vi "Ultimate Tab Control.vi"() -> ()   [LabVIEW 2020]
panel:
  in  "button name (\"OK\")":string
  in  "stop":bool
  in  "Page 5":bool
  in  "Radio Buttons":enum32{"Page 1", "Page 2", "Page 3", "Page 4"}(radio)=enum."Page 3"
  in  "Tab Control":T1(tab)
  in  "DOWN":bool
  in  "UP":bool
  out "DOWN":bool
  out "UP":bool
  in  "Rotation":enum32{"Left", "Neutral", "Right"}(radio)=enum."Neutral"
  in  "Slide":dbl(slide) scale=0.0..10.0
  out "Gauge":dbl(knob) scale=0.0..10.0
  in  "PRESS":bool
  out "Waveform Chart":dbl(graph)=1.524663471811628
  # "Notice that the stop button\nis under shadowed.\nThis means it is common to\nall pages of the tab control.\n\nIf it only needs to be visible \non three of the pages use a\nvisibility property node on the block diagram and place a constant true or false on each page."
  # "IF YOU NOTICE THE NEXT\nTIME YOU ARE IN EDIT MODE\nTHAT THE RADIO BUTTONS\nDO NOT CONTROL THE TABS.\n\nTHIS MEANS IN EDIT MODE, MAKE THE \nTABS FOR THE CONTROL VISIBLE\nIN ORDER TO TAB THROUGH THE PAGES."
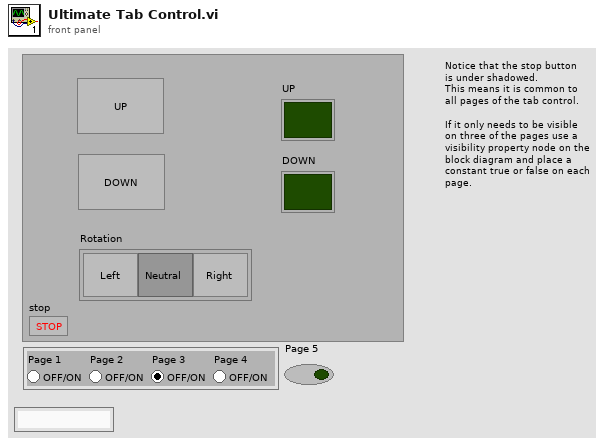
[diagram p1: front panel]
types:
  T1 = enum32{"Page 1", "Page 2", "Page 3", "Page 4", "Page 5"}
  T2 = enum8{"Enabled", "Disabled", "Disabled and Grayed Out"}
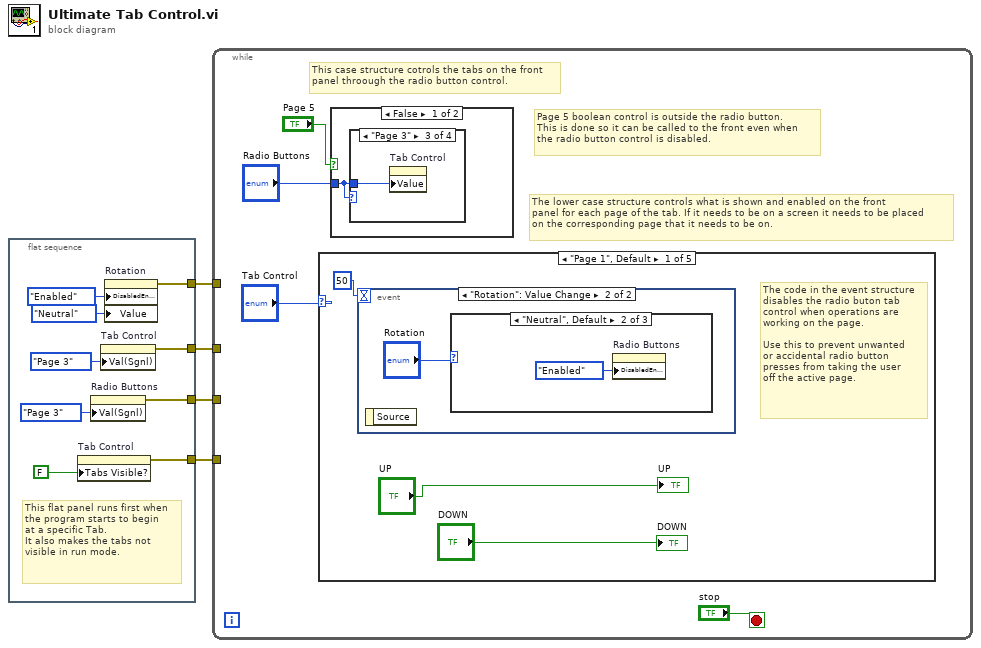
[diagram p0: block diagram]
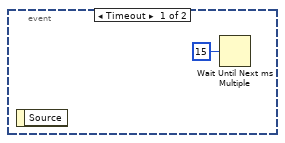
[diagram p2: hidden frame]
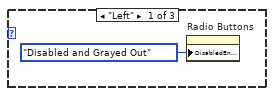
[diagram p3: hidden frame]
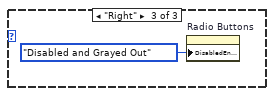
[diagram p4: hidden frame]
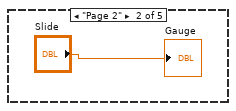
[diagram p5: hidden frame]
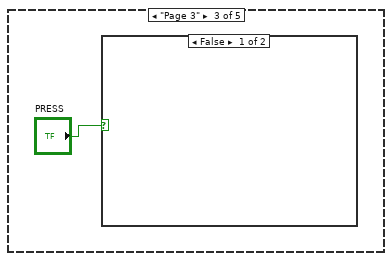
[diagram p6: hidden frame]
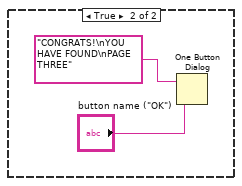
[diagram p7: hidden frame]
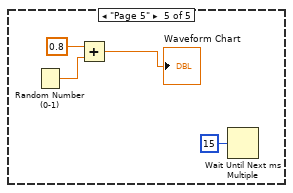
[diagram p9: hidden frame]
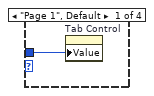
[diagram p10: hidden frame]
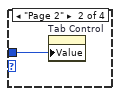
[diagram p11: hidden frame]
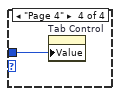
[diagram p12: hidden frame]
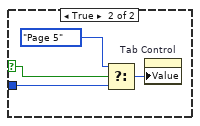
[diagram p13: hidden frame]
diagram:
  n1 = flat-sequence {
    tunnel: [w12] -> w4
    tunnel: [w10] -> w3
    tunnel: [w8] -> w2
    tunnel: [w6] -> w1
    frame #0 {
      # "This flat panel runs first when\nthe program starts to begin\nat a specific Tab.\nIt also makes the tabs not \nvisible in run mode."
      n2 = property on="Tab Control" class="TabCtl (strict)"("Tabs Visible?"=FALSE) -> (error out=w8:errorcluster)  [unwired: 2 in, 1 out]
      n3 = property on="Radio Buttons" class="RadioBtnsControl (strict)"("Val(Sgnl)"=enum32{"Page 1", "Page 2", "Page 3", "Page 4"}."Page 3" ("Value (Signaling)")) -> (error out=w10:errorcluster)  [unwired: 2 in, 1 out]
      n4 = property on="Tab Control" class="TabCtl (strict)"("Val(Sgnl)"=T1."Page 3" ("Value (Signaling)")) -> (error out=w12:errorcluster)  [unwired: 2 in, 1 out]
      n5 = property on="Rotation" class="RadioBtnsControl (strict)"("DisabledEnum"=T2."Enabled" ("Disabled"), "Value"=enum32{"Left", "Neutral", "Right"}."Neutral" ("Value (Signaling)")) -> (error out=w6:errorcluster)  [unwired: 2 in, 1 out]
    }
  }
  n6 = while {
    tunnel: w4 -> [_]
    tunnel: w3 -> [_]
    tunnel: w2 -> [_]
    tunnel: w1 -> [_]
    stop <- "stop" stop-if-true
    # "The lower case structure controls what is shown and enabled on the front\npanel for each page of the tab. If it needs to be on a screen it needs to be placed\non the corresponding page that it needs to be on."
    # "Page 5 boolean control is outside the radio button.\nThis is done so it can be called to the front even when\nthe radio button control is disabled."
    # "This case structure cotrols the tabs on the front\npanel throough the radio button control."
    n7 = case shown="\"Page 1\", Default" "Tab Control" {
      frame "Page 1", Default {
        # "The code in the event structure\ndisables the radio buton tab\ncontrol when operations are\nworking on the page.\n\nUse this to prevent unwanted \nor accidental radio button\npresses from taking the user\noff the active page."
        n8 = event shown="[1] \"Rotation\": Value Change" {
          selector: _ -> [_ _]
          dyn-events: _ -> [_ _]
          timeout: 50 -> [_ _]
          event Timeout {
            n9 = event-data() -> ()  [unwired: 1 in, 1 out]
            n10 = Wait Until Next ms Multiple(millisecond multiple=u32 15) -> ()  [unwired: 1 out]
          }
          event "Rotation": Value Change {
            n11 = event-data() -> ()  [unwired: 1 in, 1 out]
            n12 = case shown="\"Neutral\", Default" "Rotation" {
              frame "Left" {
                n13 = property on="Radio Buttons" class="RadioBtnsControl (strict)"("DisabledEnum"=T2."Disabled and Grayed Out" ("Disabled")) -> ()  [unwired: 2 in, 2 out]
              }
              frame "Neutral", Default {
                n14 = property on="Radio Buttons" class="RadioBtnsControl (strict)"("DisabledEnum"=T2."Enabled" ("Disabled")) -> ()  [unwired: 2 in, 2 out]
              }
              frame "Right" {
                n15 = property on="Radio Buttons" class="RadioBtnsControl (strict)"("DisabledEnum"=T2."Disabled and Grayed Out" ("Disabled")) -> ()  [unwired: 2 in, 2 out]
              }
            }
          }
        }
        "DOWN" <- "DOWN"
        "UP" <- "UP"
      }
      frame "Page 2" {
        "Gauge" <- "Slide"
      }
      frame "Page 3" {
        n16 = case shown="False" "PRESS" {
          frame False {
          }
          frame True {
            n17 = One Button Dialog(message="CONGRATS!\nYOU HAVE FOUND\nPAGE THREE", button name ("OK")="button name (\"OK\")") -> ()  [unwired: 1 out]
          }
        }
      }
      frame "Page 4" {
        # "TEXT BOX"
      }
      frame "Page 5" {
        n18 = Random Number (0-1)() -> (number: 0 to 1=w32:dbl)
        n19 = Add(x=0.8, y=w32) -> (x+y=→"Waveform Chart":dbl)
        n20 = Wait Until Next ms Multiple(millisecond multiple=u32 15) -> ()  [unwired: 1 out]
      }
    }
    n21 = case shown="False" "Page 5" {
      selector: "Page 5" -> [_ w40]
      tunnel: "Radio Buttons" -> [w34 w39]
      frame False {
        n22 = case shown="\"Page 3\"" w34 {
          tunnel: w34 -> [w35 w36 w37 w38]
          frame "Page 1", Default {
            n23 = property on="Tab Control" class="TabCtl (strict)"("Value"=w35) -> ()  [unwired: 2 in, 2 out]
          }
          frame "Page 2" {
            n24 = property on="Tab Control" class="TabCtl (strict)"("Value"=w36) -> ()  [unwired: 2 in, 2 out]
          }
          frame "Page 3" {
            n25 = property on="Tab Control" class="TabCtl (strict)"("Value"=w37) -> ()  [unwired: 2 in, 2 out]
          }
          frame "Page 4" {
            n26 = property on="Tab Control" class="TabCtl (strict)"("Value"=w38) -> ()  [unwired: 2 in, 2 out]
          }
        }
      }
      frame True {
        n27 = Select(t=T1."Page 5" ("Tab Control"), s=w40, f=w39) -> (s? t:f=w41:T1)
        n28 = property on="Tab Control" class="TabCtl (strict)"("Value"=w41) -> ()  [unwired: 2 in, 2 out]
      }
    }
  }
